vi "Set Parameter Value by Name.vi"(0 "Parameter Array":string[](array[string]), 7 "Parameter Name":string, 9 "flattened value":string, 12 "Create if not found":bool, 13 "Override if found":bool=TRUE) -> (4 "Parameter Array Out":string[](array[string]), 6 "Value is there":bool, 8 "Found?":bool, 10 "Created New":bool)   [LabVIEW 2014]
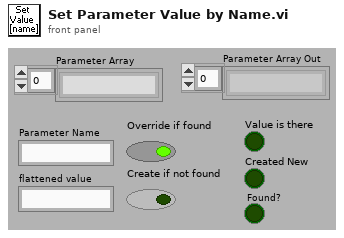
[diagram p1: front panel]
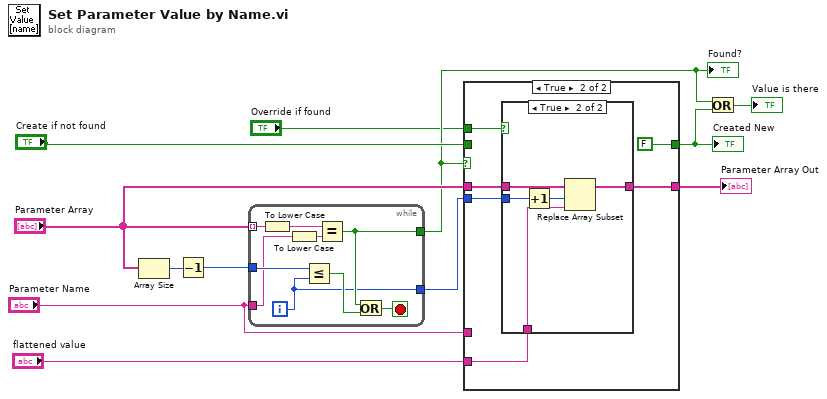
[diagram p0: block diagram]
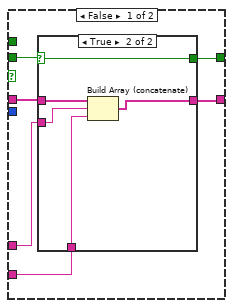
[diagram p2: hidden frame]
diagram:
  n1 = Array Size(array="Parameter Array") -> (size(s)=w9:i32)
  n2 = Decrement(x=w9) -> (x-1=w10:i32)
  n3 = while {
    tunnel: "Parameter Array" -> [w20] mode=indexing
    tunnel: w10 -> [w21]
    tunnel: "Parameter Name" -> [w19]
    tunnel: [w14] -> w4
    tunnel: [w13] -> w11
    i -> [w13]
    stop <- w18 stop-if-true
    n4 = To Lower Case(string=w20) -> (all lower case string=w16:string)
    n5 = To Lower Case(string=w19) -> (all lower case string=w15:string)
    n6 = Less Or Equal?(x=w21, y=w13) -> (x <= y?=w17:bool)
    n7 = Equal?(x=w16, y=w15) -> (x = y?=w14:bool)
    n8 = Or(x=w14, y=w17) -> (x .or. y?=w18:bool)
  }
  "Found?" <- w4
  n9 = case shown="True" w4 {
    tunnel: w11 -> [_ w38]
    tunnel: "Parameter Array" -> [w27 w40]
    tunnel: [w24 w39] -> w7
    tunnel: "flattened value" -> [w25 w37]
    tunnel: "Create if not found" -> [w23 _]
    tunnel: "Parameter Name" -> [w26 _]
    tunnel: [w22 FALSE] -> w3
    tunnel: "Override if found" -> [_ w35]
    frame False {
      n10 = case shown="True" w23 {
        selector: w23 -> [w28 w30]
        tunnel: w27 -> [w29 w34]
        tunnel: [w29 w31] -> w24
        tunnel: w25 -> [_ w33]
        tunnel: w26 -> [_ w32]
        tunnel: [w28 w30] -> w22
        frame False {
        }
        frame True {
          n11 = Build Array (concatenate)(w34, w32, w33) -> (w31:string[])
        }
      }
    }
    frame True {
      n12 = case shown="True" w35 {
        tunnel: w40 -> [w41 w46]
        tunnel: [w41 w45] -> w39
        tunnel: w38 -> [_ w44]
        tunnel: w37 -> [_ w43]
        frame False {
        }
        frame True {
          n13 = Increment(x=w44) -> (x+1=w42:i32)
          n14 = Replace Array Subset(array=w46, new element=w43, index=w42) -> (w45:string[])
        }
      }
    }
  }
  "Parameter Array Out" <- w7
  "Created New" <- w3
  n15 = Or(x=w4, y=w3) -> (x .or. y?=→"Value is there":bool)
